vi "control_label_transparent.vi"(8 "error in (no error)":errorcluster, 11 "VI Ref In":refnum<vi>) -> (0 "error out":errorcluster, 3 "VI Ref Out":refnum<vi>)   [LabVIEW 2018]
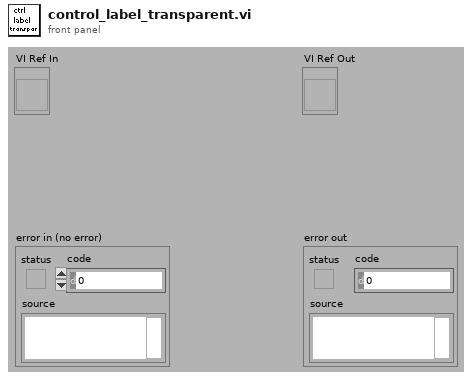
[diagram p1: front panel]
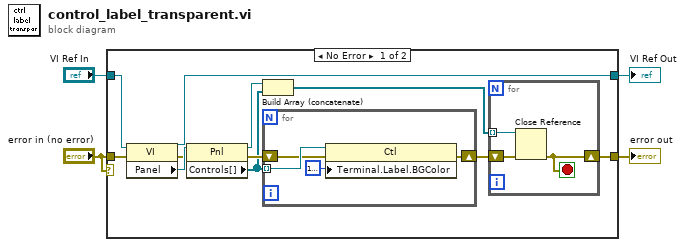
[diagram p0: block diagram]
diagram:
  n1 = case shown="No Error" "error in (no error)" {
    tunnel: [w8 w24] -> w4
    tunnel: "VI Ref In" -> [w7 w24]
    tunnel: "error in (no error)" -> [w6 w23]
    tunnel: [w5 w23] -> w2
    frame No Error {
      n2 = property class="VI"(reference=w7, error in=w6) -> (reference out=w8:refnum<vi>, error out=w14:errorcluster, "Panel"=w15:refnum<vi>)
      n3 = property class="Pnl"(reference=w15, error in=w14) -> (reference out=w12:refnum<vi>, error out=w13:errorcluster, "Controls[]"=w11:refnum<vi>[])
      n4 = Build Array (concatenate)(w12, w11) -> (w10:refnum<vi>[])
      n5 = for {
        tunnel: w11 -> [w22] mode=indexing
        shift-right: [w19] -> w9
        shift-left: w13 -> [w21]
        n6 = property class="Ctl"(reference=w22, error in=w21, "Terminal.Label.BGColor"=u32 16777216) -> (error out=w19:errorcluster)  [unwired: 1 out]
      }
      n7 = for {
        tunnel: w10 -> [w18] mode=indexing
        shift-right: [w16] -> w5
        shift-left: w9 -> [w17]
        stop <- w16 stop-if-true
        n8 = Close Reference(reference=w18, error in (no error)=w17) -> (error out=w16:errorcluster)
      }
    }
    frame Error {
    }
  }
  "VI Ref Out" <- w4
  "error out" <- w2
